vi "sv_Change Base Length Unit.vi"(5 "desired base units for vibration":i32(ring) items=["no change"=-1, "g"=386, "m"=0, "cm"=4, "mm"=2, "micron"=3, "in"=1, "mil"=5], 7 "custom label in":string="EU", 8 "engineering units in":T1=3 items=["custom..."=0, "V"=1, "A"=21, "C"=30, "pC"=31, "s"=32, "-"=29, "Pa"=2, "N"=20, "g"=3, "m/s^2"=4, "m/s"=5, "m"=6, "mm/s"=12, "mm"=13, "micron/s"=14, "micron"=15, "in/s^2"=7, "in/s"=8, "in"=9, "mil/s"=10, "mil"=11, "rad/s^2"=16, "rad/s"=17, "rad"=18, "deg/s^2"=26, "deg/s"=27, "deg"=28, "RPM"=22, "cycle/s^2"=23, "Hz"=24, "cycle"=25, "strain"=19], 9 "value in [EU]":dbl=1.0) -> (1 "custom label out":string="m/s^2", 2 "engineering units out":T1=4 items=["custom..."=0, "V"=1, "A"=21, "C"=30, "pC"=31, "s"=32, "-"=29, "Pa"=2, "N"=20, "g"=3, "m/s^2"=4, "m/s"=5, "m"=6, "mm/s"=12, "mm"=13, "micron/s"=14, "micron"=15, "in/s^2"=7, "in/s"=8, "in"=9, "mil/s"=10, "mil"=11, "rad/s^2"=16, "rad/s"=17, "rad"=18, "deg/s^2"=26, "deg/s"=27, "deg"=28, "RPM"=22, "cycle/s^2"=23, "Hz"=24, "cycle"=25, "strain"=19], 3 "value out [desired EU]":dbl=9.80665 format="%#_9g")   [LabVIEW 2017]
uses:
  <vilib>/addons/_NISVFA/_Shared subVIs/Controls/svc_Engineering Units Text Ring.ctl
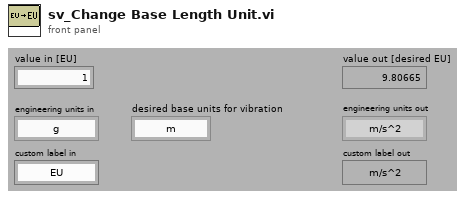
[diagram p1: front panel]
types:
  T1 = typedef "svc_Engineering Units Text Ring.ctl" = u16
  T2 = enum16{"custom...", "V", "Pa", "g", "m/s^2", "m/s", "m", "in/s^2", "in/s", "in", "mil/s", "mil", "mm/s", "mm", "micron/s", "micron", "rad/s^2", "rad/s", "rad", "strain", "N", "A", "rpm", "cycle/s^2", "Hz", "cycle", "deg/s^2", "deg/s", "deg", "Undefined"}
  T3 = enum16{"custom...", "V", "Pa", "g", "m/s^2", "m/s", "m", "in/s^2", "in/s", "in", "mil/s", "mil", "mm/s", "mm", "micron/s", "micron", "rad/s^2", "rad/s", "rad", "strain", "N", "A", "rpm", "cycle/s^2", "Hz", "cycle", "deg/s^2", "deg/s", "deg", "Undefined", "C", "pC"}
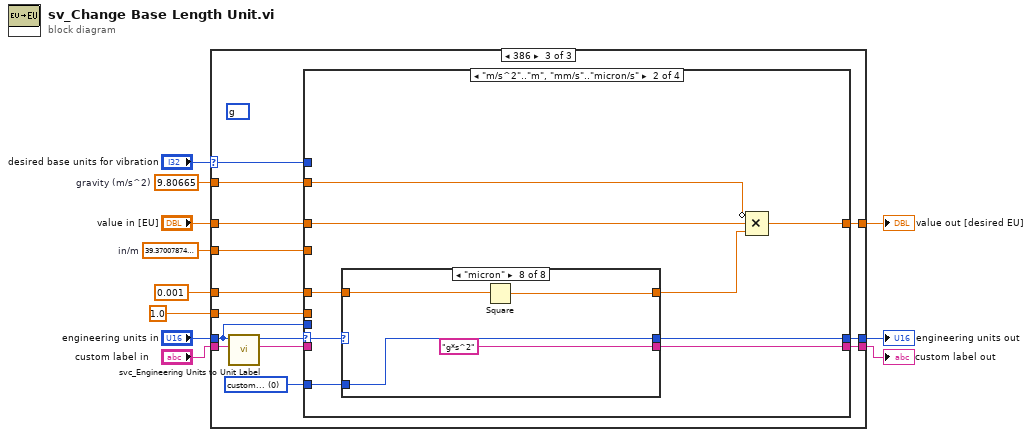
[diagram p0: block diagram]
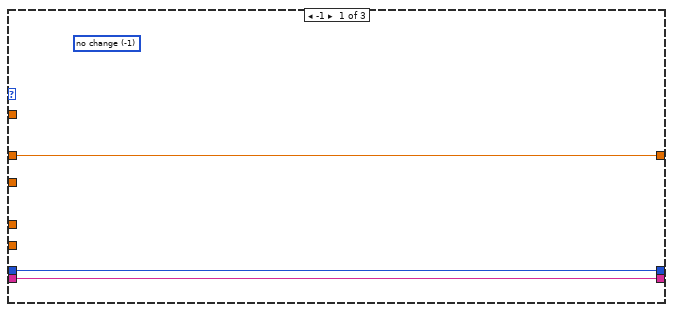
[diagram p2: hidden frame]
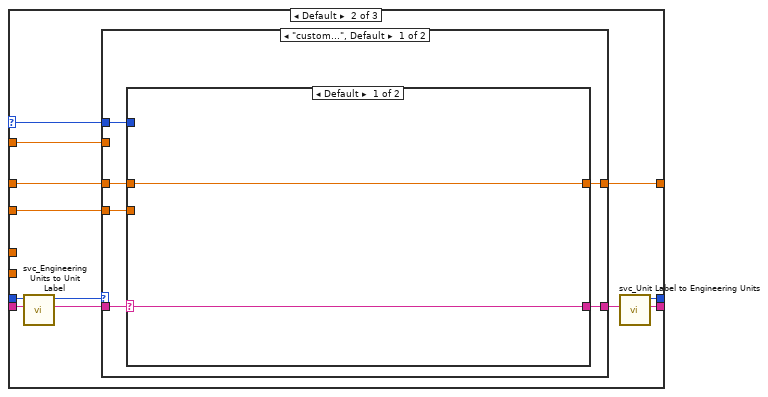
[diagram p3: hidden frame]
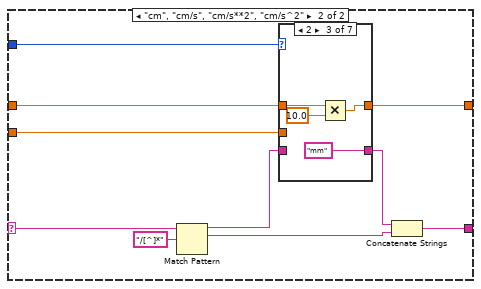
[diagram p4: hidden frame]
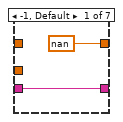
[diagram p5: hidden frame]
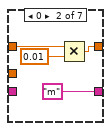
[diagram p6: hidden frame]
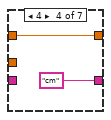
[diagram p7: hidden frame]
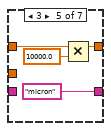
[diagram p8: hidden frame]
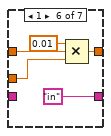
[diagram p9: hidden frame]
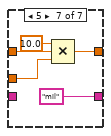
[diagram p10: hidden frame]
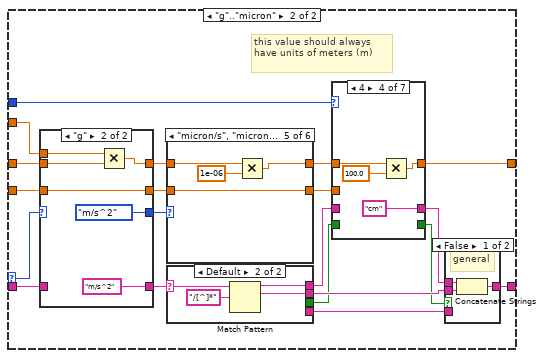
[diagram p11: hidden frame]
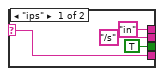
[diagram p13: hidden frame]
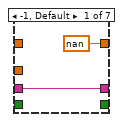
[diagram p15: hidden frame]
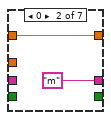
[diagram p16: hidden frame]
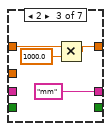
[diagram p17: hidden frame]
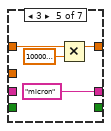
[diagram p18: hidden frame]
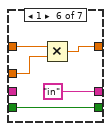
[diagram p19: hidden frame]
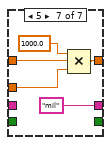
[diagram p20: hidden frame]
diagram:
  w3 = 39.37007874015748  # in/m
  w6 = 9.80665  # gravity (m/s^2)
  n1 = case shown="386" "desired base units for vibration" {
    selector: "desired base units for vibration" -> [_ w21 w169]
    tunnel: [w14 w26 w171] -> w11
    tunnel: "engineering units in" -> [w13 w25 w162]
    tunnel: "value in [EU]" -> [w14 w24 w170]
    tunnel: [w13 w22 w164] -> w8
    tunnel: w6 -> [_ w18 w166]
    tunnel: "custom label in" -> [w12 w17 w165]
    tunnel: [w12 w16 w163] -> w4
    tunnel: w3 -> [_ w15 w161]
    tunnel: 0.001 -> [_ _ w160]
    tunnel: 1.0 -> [_ _ w158]
    frame -1 {
      (unwired) -1 items=["no change"=-1, "g"=386, "m"=0, "cm"=4, "mm"=2, "microns"=3, "in"=1, "mils"=5] ("desired base units for vibration")
    }
    frame Default {
      n2 = call <vilib>:"svc_Engineering Units to Unit Label.vi"("custom label"=w17, "engineering units"=w25) -> ("unit label"=w20:string, "engineering units enum"=w19:T3)  [unwired: 8 in]
      n3 = case shown="\"custom...\", Default" w19 {
        selector: w19 -> [_ w79]
        tunnel: [w30 w90] -> w26
        tunnel: w24 -> [w31 w88]
        tunnel: [w29 w82] -> w23
        tunnel: w21 -> [w28 w81]
        tunnel: w20 -> [w32 w80]
        tunnel: w18 -> [_ w78]
        tunnel: w15 -> [w27 w73]
        frame "custom...", Default {
          n4 = case shown="Default" w32 {
            selector: w32 -> [w33 w39]
            tunnel: w31 -> [w34 w37]
            tunnel: [w34 w35] -> w30
            tunnel: [w33 w38] -> w29
            tunnel: w28 -> [_ w40]
            tunnel: w27 -> [_ w36]
            frame Default {
            }
            frame "cm", "cm/s", "cm/s**2", "cm/s^2" {
              n5 = Match Pattern(string=w39, regular expression="/[^]*") -> (before substring=w43:string, match substring=w42:string)  [unwired: 1 in, 2 out]
              n6 = case shown="2" w40 {
                tunnel: [nan ("unit (none)") w47 w51 w55 w58 w63 w68] -> w35
                tunnel: w37 -> [_ w49 w53 w55 w59 w64 w69]
                tunnel: w43 -> [w46 _ _ _ _ _ _]
                tunnel: [w46 "m" "mm" "cm" "micron" "in" "mil"] -> w41
                tunnel: w36 -> [_ _ _ _ _ w62 w67]
                frame -1, Default {
                }
                frame 0 {
                  n7 = Multiply(x=w49, y=0.01) -> (x*y=w47:dbl)
                }
                frame 2 {
                  n8 = Multiply(x=w53, y=10.0) -> (x*y=w51:dbl)
                }
                frame 4 {
                }
                frame 3 {
                  n9 = Multiply(x=w59, y=10000.0) -> (x*y=w58:dbl)
                }
                frame 1 {
                  n10 = Compound Arithmetic op=MULTIPLY(0.01 ("value"), w64, w62) -> (w63:dbl)
                }
                frame 5 {
                  n11 = Compound Arithmetic op=MULTIPLY(10.0 ("value"), w69, w67) -> (w68:dbl)
                }
              }
              n12 = Concatenate Strings(w41, w42) -> (w38:string)
            }
          }
        }
        frame "g".."micron" {
          # "this value should always have units of meters (m)"
          n13 = case shown="\"g\"" w79 {
            selector: w79 -> [w106 _]
            tunnel: [w106 T2."m/s^2" ("engineering units enum")] -> w86
            tunnel: w88 -> [w105 w112]
            tunnel: [w105 w111] -> w87
            tunnel: w80 -> [w104 _]
            tunnel: [w104 "m/s^2" ("unit label")] -> w77
            tunnel: w78 -> [_ w109]
            tunnel: w73 -> [w103 w107]
            tunnel: [w103 w107] -> w72
            frame Default {
            }
            frame "g" {
              n14 = Multiply(x=w109, y=w112) -> (x*y=w111:dbl)
            }
          }
          n15 = case shown="\"micron/s\", \"micron\"" w86 {
            tunnel: w87 -> [w139 w142 w147 w150 w154 _]
            tunnel: [w139 w141 w144 w149 w153 nan ("value in [EU]")] -> w89
            tunnel: [w140 w143 w145 w151 w155 w157] -> w71
            tunnel: w72 -> [w140 w143 w145 w151 w155 w157]
            frame "m/s^2".."m" {
            }
            frame "in/s^2".."in" {
              n16 = Divide(x=w142, y=w143) -> (x/y=w141:dbl)
            }
            frame "mil/s", "mil" {
              n17 = Compound Arithmetic op=MULTIPLY(w147, invert w145, 0.001) -> (w144:dbl)
            }
            frame "mm/s", "mm" {
              n18 = Multiply(x=w150, y=0.001) -> (x*y=w149:dbl)
            }
            frame "micron/s", "micron" {
              n19 = Multiply(x=w154, y=1e-06) -> (x*y=w153:dbl)
            }
            frame Default {
            }
          }
          n20 = case shown="Default" w77 {
            selector: w77 -> [w95 w99]
            tunnel: ["in" w101] -> w85
            tunnel: ["/s" w100] -> w84
            tunnel: [TRUE _] -> w76
            tunnel: [w95 _] -> w74
            frame "ips" {
            }
            frame Default {
              n21 = Match Pattern(string=w99, regular expression="/[^]*") -> (before substring=w101:string, match substring=w100:string)  [unwired: 1 in, 2 out]
            }
          }
          n22 = case shown="4" w81 {
            tunnel: [nan ("value in [EU]") w115 w117 w121 w126 w129 w138] -> w90
            tunnel: w89 -> [_ w115 w119 w123 w127 w131 w136]
            tunnel: w85 -> [w114 _ _ _ _ _ _]
            tunnel: [w114 "m" "mm" "cm" "micron" "in" "mil"] -> w83
            tunnel: w76 -> [_ _ _ _ _ w132 _]
            tunnel: [_ _ _ _ _ w132 _] -> w75
            tunnel: w71 -> [_ _ _ _ _ w130 w134]
            frame -1, Default {
            }
            frame 0 {
            }
            frame 2 {
              n23 = Multiply(x=w119, y=1000.0) -> (x*y=w117:dbl)
            }
            frame 4 {
              n24 = Multiply(x=w123, y=100.0) -> (x*y=w121:dbl)
            }
            frame 3 {
              n25 = Multiply(x=w127, y=1000000.0) -> (x*y=w126:dbl)
            }
            frame 1 {
              n26 = Multiply(x=w131, y=w130) -> (x*y=w129:dbl)
            }
            frame 5 {
              n27 = Compound Arithmetic op=MULTIPLY(1000.0, w136, w134) -> (w138:dbl)
            }
          }
          n28 = case shown="False" w75 {
            tunnel: w84 -> [w93 _]
            tunnel: w83 -> [w92 _]
            tunnel: [w91 w94] -> w82
            tunnel: w74 -> [_ w94]
            frame False {
              # "general"
              n29 = Concatenate Strings(w92, w93) -> (w91:string)
            }
            frame True {
              # "ips"
            }
          }
        }
      }
      n30 = call <vilib>:"svc_Unit Label to Engineering Units.vi"("unit label"=w23) -> ("unit label out"=w16:string, "engineering units"=w22:T1)  [unwired: 9 in]
    }
    frame 386 {
      w159 = T1 0 items=["custom..."=0, "V"=1, "A"=21, "Pa"=2, "N"=20, "g"=3, "m/s^2"=4, "m/s"=5, "m"=6, "mm/s"=12, "mm"=13, "micron/s"=14, "micron"=15, "in/s^2"=7, "in/s"=8, "in"=9, "mil/s"=10, "mil"=11, "rad/s^2"=16, "rad/s"=17, "rad"=18, "deg/s^2"=26, "deg/s"=27, "deg"=28, "RPM"=22, "cycle/s^2"=23, "Hz"=24, "cycle"=25, "strain"=19] ("engineering units out")
      (unwired) 386 items=["no change"=-1, "g"=386, "m"=0, "cm"=4, "mm"=2, "microns"=3, "in"=1, "mils"=5] ("desired base units for vibration")
      n31 = call <vilib>:"svc_Engineering Units to Unit Label.vi"("custom label"=w165, "engineering units"=w162) -> ("unit label"=w168:string, "engineering units enum"=w167:T3)  [unwired: 8 in]
      n32 = case shown="\"m/s^2\"..\"m\", \"mm/s\"..\"micron/s\"" w167 {
        selector: w167 -> [_ w179 w213 _]
        tunnel: [w173 w183 w219 w243] -> w171
        tunnel: w170 -> [w173 w182 w218 w244]
        tunnel: [w174 w180 w216 w242] -> w163
        tunnel: w169 -> [_ _ _ w241]
        tunnel: w168 -> [w174 _ _ w245]
        tunnel: w166 -> [_ w178 w215 w240]
        tunnel: [w172 w181 w217 w239] -> w164
        tunnel: w162 -> [w172 _ _ w238]
        tunnel: w161 -> [_ _ w214 _]
        tunnel: w160 -> [_ w176 w210 _]
        tunnel: w159 -> [_ w177 w212 w237]
        tunnel: w158 -> [_ _ w209 _]
        frame "g" {
        }
        frame "m/s^2".."m", "mm/s".."micron/s" {
          n33 = case shown="\"micron\"" w179 {
            tunnel: [w185 w188 w190 w193 w196 w200 w203 w207] -> w181
            tunnel: [_ "g" ("unit label") "g*s" "g*s^2" "g*s" "g*s" "g*s^2" "g*s^2"] -> w180
            tunnel: w177 -> [w185 _ w190 w193 w196 w200 w203 w207]
            tunnel: w176 -> [_ _ _ _ w195 w199 w202 w206]
            tunnel: [1.0 1.0 1.0 1.0 w195 w198 w202 w205] -> w175
            frame Default {
            }
            frame "m/s^2" {
              w188 = T1 3 items=["custom..."=0, "V"=1, "A"=21, "Pa"=2, "N"=20, "g"=3, "m/s^2"=4, "m/s"=5, "m"=6, "mm/s"=12, "mm"=13, "micron/s"=14, "micron"=15, "in/s^2"=7, "in/s"=8, "in"=9, "mil/s"=10, "mil"=11, "rad/s^2"=16, "rad/s"=17, "rad"=18, "deg/s^2"=26, "deg/s"=27, "deg"=28, "RPM"=22, "cycle/s^2"=23, "Hz"=24, "cycle"=25, "strain"=19] ("engineering units in")
            }
            frame "m/s" {
            }
            frame "m" {
            }
            frame "mm/s" {
            }
            frame "micron/s" {
              n34 = Square(x=w199) -> (x^2=w198:dbl)
            }
            frame "mm" {
            }
            frame "micron" {
              n35 = Square(x=w206) -> (x^2=w205:dbl)
            }
          }
          n36 = Compound Arithmetic op=MULTIPLY(invert w178, w182, w175) -> (w183:dbl)
        }
        frame "in/s^2".."mil" {
          n37 = case shown="\"in\"" w213 {
            tunnel: [w221 w224 w226 w229 w232 w235] -> w217
            tunnel: [_ "g" ("unit label") "g*s" ("unit label") "g*s^2" ("unit label") "g*s" ("unit label") "g*s^2" ("unit label")] -> w216
            tunnel: w212 -> [w221 _ w226 w229 w232 w235]
            tunnel: [w220 w222 w225 w228 w231 w234] -> w211
            tunnel: w210 -> [_ _ _ _ w231 w234]
            tunnel: w209 -> [w220 w222 w225 w228 _ _]
            frame Default {
            }
            frame "in/s^2" {
              w224 = T1 3 items=["custom..."=0, "V"=1, "A"=21, "Pa"=2, "N"=20, "g"=3, "m/s^2"=4, "m/s"=5, "m"=6, "mm/s"=12, "mm"=13, "micron/s"=14, "micron"=15, "in/s^2"=7, "in/s"=8, "in"=9, "mil/s"=10, "mil"=11, "rad/s^2"=16, "rad/s"=17, "rad"=18, "deg/s^2"=26, "deg/s"=27, "deg"=28, "RPM"=22, "cycle/s^2"=23, "Hz"=24, "cycle"=25, "strain"=19] ("engineering units in")
            }
            frame "in/s" {
            }
            frame "in" {
            }
            frame "mil/s" {
            }
            frame "mil" {
            }
          }
          n38 = Compound Arithmetic op=MULTIPLY(invert w215, w218, invert w214, w211) -> (w219:dbl)
        }
        frame "custom...", Default {
          n39 = case shown="Default" w245 {
            selector: w245 -> [w247 w250]
            tunnel: w244 -> [w248 w253]
            tunnel: [w248 w256] -> w243
            tunnel: [w247 w255] -> w242
            tunnel: w241 -> [_ _]
            tunnel: w240 -> [_ w252]
            tunnel: [w246 w254] -> w239
            tunnel: w238 -> [w246 _]
            tunnel: w237 -> [_ w249]
            frame Default {
            }
            frame "cm", "cm/s", "cm/s**2", "cm/s^2" {
              n40 = case shown="\"cm/s**2\", \"cm/s^2\", Default" w250 {
                tunnel: ["g*s" "g*s^2" "g"] -> w255
                tunnel: [w257 w260 w261] -> w254
                tunnel: w249 -> [w257 w260 _]
                frame "cm/s" {
                }
                frame "cm" {
                }
                frame "cm/s**2", "cm/s^2", Default {
                  w261 = T1 3 items=["custom..."=0, "V"=1, "A"=21, "Pa"=2, "N"=20, "g"=3, "m/s^2"=4, "m/s"=5, "m"=6, "mm/s"=12, "mm"=13, "micron/s"=14, "micron"=15, "in/s^2"=7, "in/s"=8, "in"=9, "mil/s"=10, "mil"=11, "rad/s^2"=16, "rad/s"=17, "rad"=18, "deg/s^2"=26, "deg/s"=27, "deg"=28, "RPM"=22, "cycle/s^2"=23, "Hz"=24, "cycle"=25, "strain"=19] ("engineering units out")
                }
              }
              n41 = Compound Arithmetic op=MULTIPLY(invert w252, w253, 0.01 ("value")) -> (w256:dbl)
            }
          }
        }
      }
    }
  }
  "value out [desired EU]" <- w11
  "engineering units out" <- w8
  "custom label out" <- w4
